vi "Read Carried Calories.vi"(8 "error in (no error)":errorcluster, 11 "Elf in":refnum<class "Elf.lvclass">) -> (0 "error out":errorcluster, 2 "Carried Calories":dbl, 3 "Elf out":refnum<class "Elf.lvclass">)   [LabVIEW 2017, in "Elf.lvclass"]
uses:
  Elf.lvclass
  Elf.lvclass/Elf.ctl
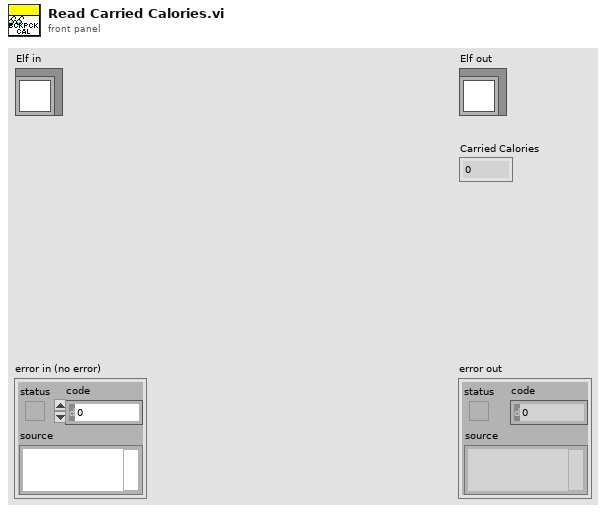
[diagram p1: front panel]
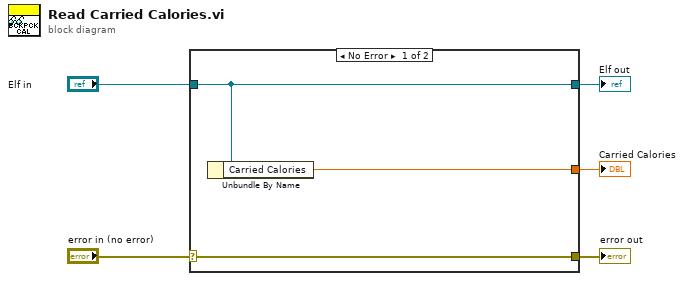
[diagram p0: block diagram]
diagram:
  n1 = case shown="No Error" "error in (no error)" {
    selector: "error in (no error)" -> [w8 w9]
    tunnel: [w8 w9] -> w4
    tunnel: [w7 w10] -> w2
    tunnel: "Elf in" -> [w7 w10]
    tunnel: [w6 _] -> w1
    frame No Error {
      n2 = Unbundle By Name(w7) -> ("Carried Calories"=w6:dbl)
    }
    frame Error {
    }
  }
  "error out" <- w4
  "Elf out" <- w2
  "Carried Calories" <- w1
